vi "testInvalidInputs.vi"(8 "error in (no error)":errorcluster, 11 "TestCase in":refnum<class "EasyXMLTest.lvclass">) -> (0 "error out":errorcluster, 3 "TestCase out":refnum<class "EasyXMLTest.lvclass">)   [LabVIEW 2013, in "EasyXMLTest.lvclass"]
doc: "Verify that error in is not overwritten"
uses:
  EasyXMLTest.lvclass
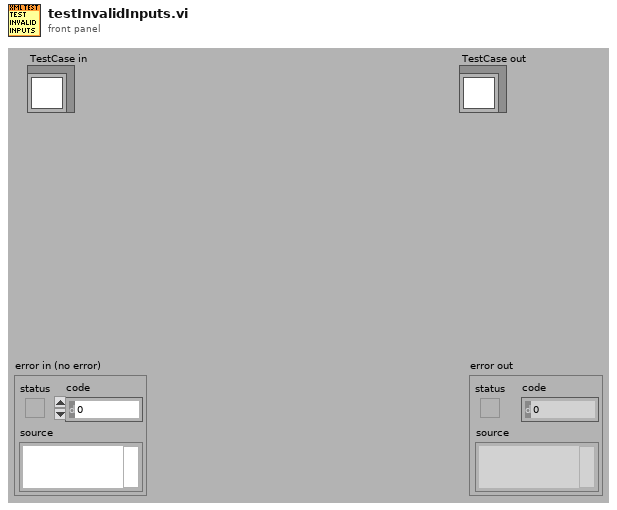
[diagram p1: front panel]
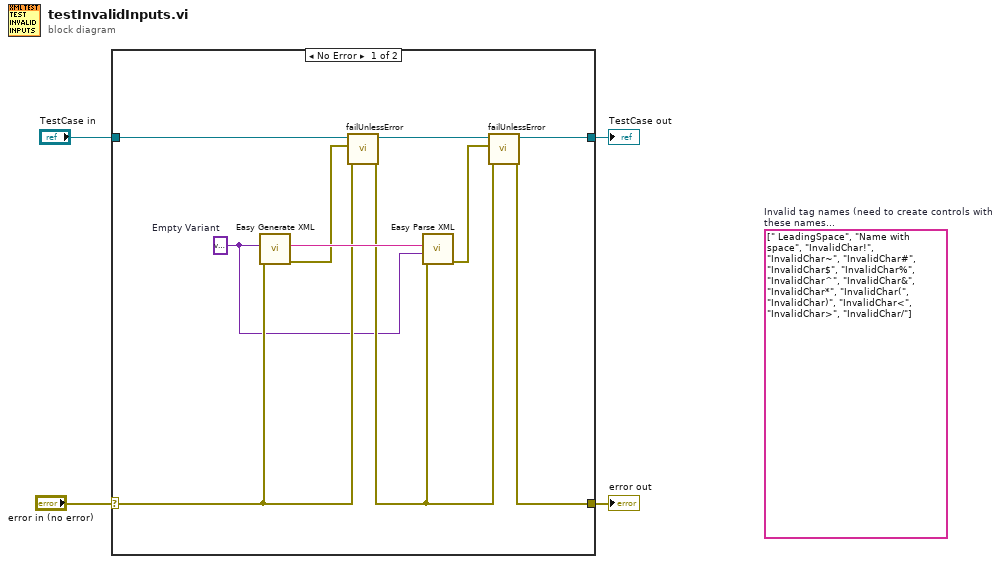
[diagram p0: block diagram]
diagram:
  (unwired) string[] [" LeadingSpace", "Name with space", "InvalidChar!", "InvalidChar~", "InvalidChar#", "InvalidChar$", "InvalidChar%", "InvalidChar^", "InvalidChar&", "InvalidChar*", "InvalidChar(", "InvalidChar)", "InvalidChar<", "InvalidChar>", "InvalidChar/"]  # Invalid tag names (need to create controls with these names...
  n1 = case shown="No Error" "error in (no error)" {
    selector: "error in (no error)" -> [w10 w16]
    tunnel: [w5 w16] -> w3
    tunnel: [w6 w15] -> w1
    tunnel: "TestCase in" -> [w14 w15]
    frame No Error {
      w7 = variant  # Empty Variant
      n2 = call "Easy Generate XML.vi"("error in (no error)"=w10, "LabVIEW Data"=w7) -> ("error out"=w11:errorcluster, "XML String"=w12:string)  [unwired: 8 in]
      n3 = call-dynamic "failUnlessError.vi"("error in (no error)"=w10, "error"=w11, "TestCase in"=w14) -> ("error out"=w8:errorcluster, "TestCase out"=w13:refnum<class "EasyXMLTest.lvclass">)  [unwired: 7 in]
      n4 = call "Easy Parse XML.vi"("error in (no error)"=w8, "LabVIEW Data (Type)"=w7, "XML String"=w12) -> ("error out"=w9:errorcluster)  [unwired: 7 in, 1 out]
      n5 = call-dynamic "failUnlessError.vi"("error in (no error)"=w8, "error"=w9, "TestCase in"=w13) -> ("error out"=w5:errorcluster, "TestCase out"=w6:refnum<class "EasyXMLTest.lvclass">)  [unwired: 7 in]
    }
    frame Error {
    }
  }
  "error out" <- w3
  "TestCase out" <- w1
